vi "Write Cell Double.vi"(0 "Report Ref In":T1, 1 "Row Index":i32, 2 "Column Index":i32, 3 "error in (no error)":errorcluster, 4 "Value":dbl) -> (5 "Report Ref Out":T1, 6 "error out":errorcluster)   [LabVIEW 2013, in "XCel Report Engine.lvlib"]
doc: "Writes a double-precision numeric value to a cell in the active worksheet.\n\nThe cell is specified by zero-based row and column coordinates. Coordinate (0, 0) corresponds to cell A1.\n\nThe value is stored as an Excel numeric value using an invariant-culture representation. NaN and positive or negative infinity are not supported and return an error.\n\nWriting the value replaces any existing cell value or formula while preserving the cell's existing formatting.\n\nThis VI is an instance of the polymorphic Write Cell.vi."
uses:
  XCel Report Engine.lvlib
  C:/Users/m.santucci/Documents/ChatGPT/LV_REPORT_ENGINE/LV/DotNet/XCelReportEngine.dll
  LV/DotNet/XCelReportEngine.dll
  Controls/Report Ref.ctl
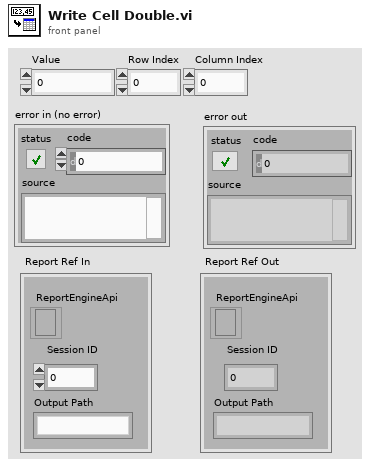
[diagram p1: front panel]
types:
  T1 = typedef "XCel Report Engine.lvlib/Report Ref.ctl" = cluster{"Session ID":i32, "Output Path":string, "ReportEngineApi":refnum<k24>}
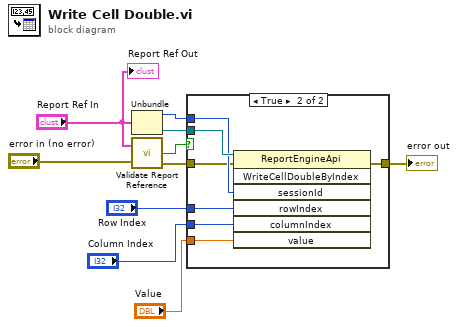
[diagram p0: block diagram]
diagram:
  n1 = Unbundle("Report Ref In") -> ("Session ID"=w8:i32, "ReportEngineApi"=w10:refnum<k24>)  [unwired: 1 out]
  n2 = call "Validate Report Reference.vi"("Report Ref In"="Report Ref In", "error in (no error)"="error in (no error)") -> ("Valid"=w1:bool, "error out"=w2:errorcluster)  [unwired: 1 out]
  n3 = case shown="True" w1 {
    tunnel: w10 -> [_ w18]
    tunnel: [w11 w17] -> w9
    tunnel: w8 -> [_ w16]
    tunnel: "Row Index" -> [_ w15]
    tunnel: "Column Index" -> [_ w14]
    tunnel: "Value" -> [_ w13]
    tunnel: w2 -> [w11 w12]
    frame False {
    }
    frame True {
      n4 = invoke class="ReportEngineApi" method="WriteCellDoubleByIndex"(reference=w18, error in=w12, "sessionId"=w16, "rowIndex"=w15, "columnIndex"=w14, "value"=w13) -> (error out=w17:errorcluster)  [unwired: 1 in, 6 out]
    }
  }
  "error out" <- w9
  "Report Ref Out" <- "Report Ref In"
